vi "Motor.vi"(5 "PID gains":T1={"proportional gain (Kc)"=5.0, "integral time (Ti, min)"=0.0, "derivative time (Td, min)"=0.0002}, 7 "Enum":T2, 8 "error in (no error)":errorcluster, 9 "Reset":bool, 10 "dt(s)":dbl, 11 "RPM":dbl) -> (0 "error out":errorcluster, 1 "process":dbl, 2 "setpoint":dbl, 3 "PWM":dbl)   [LabVIEW 2019]
uses:
  <vilib>/addons/control/pid/NI_PID_pid.lvlib
  <vilib>/addons/control/pid/pid.llb/PID (DBL).vi
  motor enum.ctl
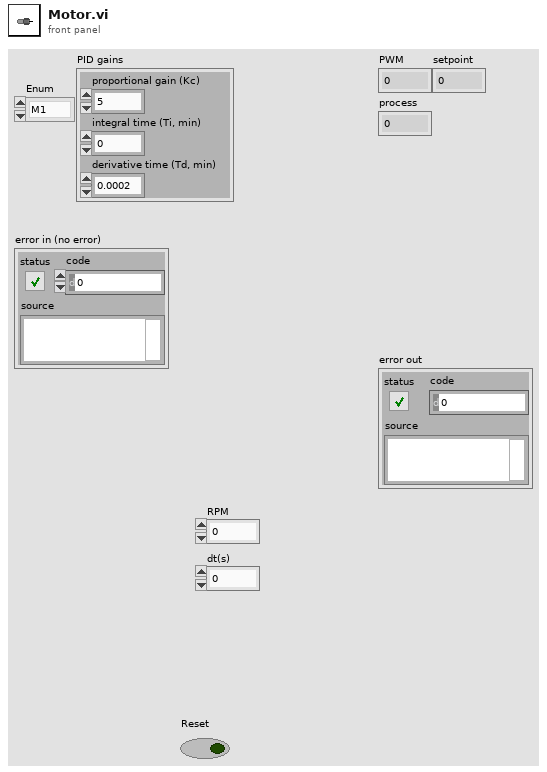
[diagram p1: front panel]
types:
  T1 = cluster{"proportional gain (Kc)":dbl, "integral time (Ti, min)":dbl, "derivative time (Td, min)":dbl}
  T2 = typedef "motor enum.ctl" = enum16{"M1", "M2", "M3", "M4"}
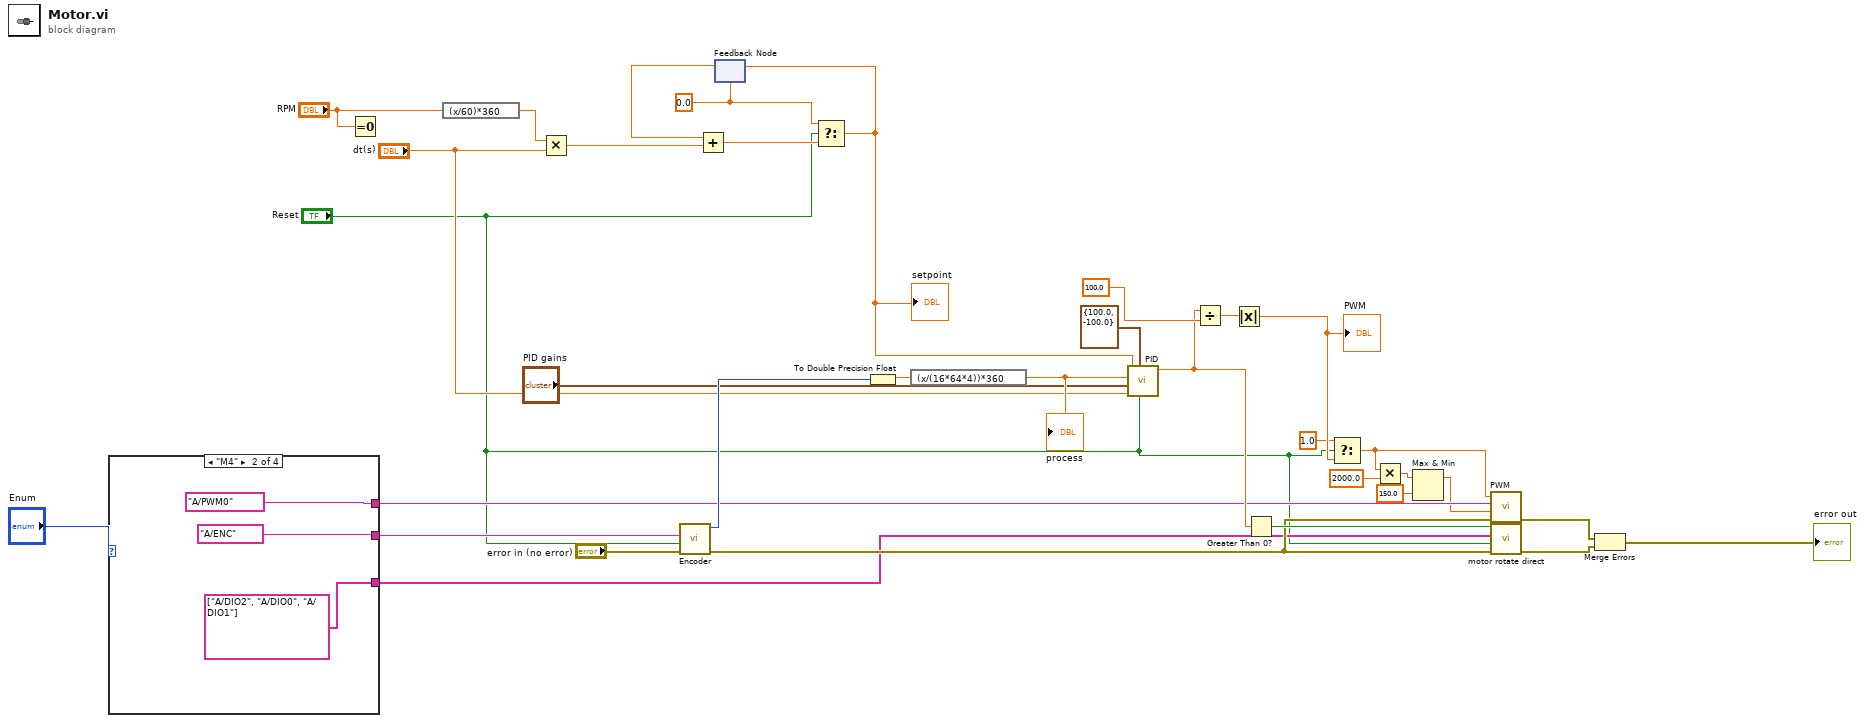
[diagram p0: block diagram]
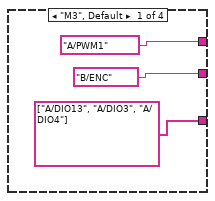
[diagram p2: hidden frame]
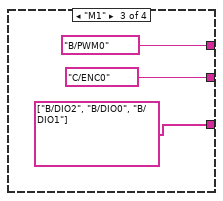
[diagram p3: hidden frame]
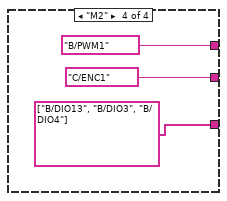
[diagram p4: hidden frame]
diagram:
  w21 = 0.0
  n1 = case shown="\"M4\"" "Enum" {
    tunnel: [tag "B/ENC" ("Channel Name") tag "A/ENC" ("Channel Name") tag "C/ENC0" ("Channel Name") tag "C/ENC1" ("Channel Name")] -> w24
    tunnel: [tag[] ["A/DIO13", "A/DIO3", "A/DIO4"] ("Channel Names") tag[] ["A/DIO2", "A/DIO0", "A/DIO1"] ("Channel Names") tag[] ["B/DIO2", "B/DIO0", "B/DIO1"] ("Channel Names") tag[] ["B/DIO13", "B/DIO3", "B/DIO4"] ("Channel Names")] -> w15
    tunnel: [tag "A/PWM1" ("Channel Name") tag "A/PWM0" ("Channel Name") tag "B/PWM0" ("Channel Name") tag "B/PWM1" ("Channel Name")] -> w14
    frame "M3", Default {
    }
    frame "M4" {
    }
    frame "M1" {
    }
    frame "M2" {
    }
  }
  n2 = Equal To 0?(x="RPM") -> ()  [unwired: 1 out]
  n3 = expression code="(x/60)*360"("RPM") -> (w33:dbl)
  n4 = Multiply(x=w33, y="dt(s)") -> (x*y=w32:dbl)
  n5 = call "Encoder.vi"("error in (no error)"="error in (no error)", "Reset Counter"="Reset", "Channel Name"=w24) -> ("error out"=w16:errorcluster, "Counter Value"=w30:i32)  [unwired: 6 in, 1 out]
  n6 = feedback #1(w21) -> (w31:dbl)
  n7 = Add(x=w31, y=w32) -> (x+y=w23:dbl)
  n8 = Select(t=w21, s="Reset", f=w23) -> (s? t:f=w22:dbl)
  "setpoint" <- w22
  n9 = feedback-in #1(w22) -> ()
  n10 = To Double Precision Float(number=w30) -> (double precision float=w29:dbl)
  n11 = expression code="(x/(16*64*4))*360"(w29) -> (w28:dbl)
  "process" <- w28
  n12 = call-poly <vilib>:"PID.vi"("reinitialize? (F)"="Reset", "output range"=cluster{"output high":dbl, "output low":dbl} {"output high"=100.0, "output low"=-100.0}, "dt (s)"="dt(s)", "PID gains"="PID gains", "process variable"=w28, "setpoint"=w22) -> ("output"=w18:dbl)  [unwired: 4 in, 1 out]
  n13 = Divide(x=w18, y=100.0 ("output high")) -> (x/y=w19:dbl)
  n14 = Absolute Value(x=w19) -> (abs(x)=w8:dbl)
  "PWM" <- w8
  n15 = Greater Than 0?(x=w18) -> (x > 0?=w17:bool)
  n16 = Select(t=1.0, s="Reset", f=w8) -> (s? t:f=w5:dbl)
  n17 = Multiply(x=w5, y=2000.0) -> (x*y=w3:dbl)
  n18 = Max & Min(x=w3, y=150.0) -> (max(x,y)=w1:dbl)  [unwired: 1 out]
  n19 = call "PWM.vi"("error in (no error)"=w16, "Frequency [Hz]"=w1, "Channel Name"=w14, "Duty Cycle"=w5) -> ("error out"=w12:errorcluster)  [unwired: 7 in]
  n20 = call "motor rotate direct.vi"("error in (no error)"=w16, "RESET"="Reset", "Channel Names"=w15, "Boolean"=w17) -> ("error out"=w13:errorcluster)  [unwired: 7 in]
  n21 = Merge Errors(w12, w13) -> (→"error out":errorcluster)
